vi "Invalid Iteration Error.vi"(7 "error source vi name":string, 8 "error in (no error)":errorcluster, 9 "expected iteration":u64, 10 "actual iteration":u64, 11 "Transfer Group in":refnum<class "Transfer Group.lvclass">) -> (0 "error out":errorcluster, 3 "Transfer Group out":refnum<class "Transfer Group.lvclass">)   [LabVIEW 2017, in "DSF Core.lvlib" / "Transfer Group.lvclass"]
uses:
  Transfer Group.lvclass
  Errors.ctl
  Transfer Group.lvclass/Transfer Group.ctl
  <vilib>/NI/Memory Manager/VIs/New Error Cluster (512B).vi
  <vilib>/NI/Memory Manager/VIs/Write Numeric Scalar to Source (Base10 U64).vi
  Framework/Engine Library Name.vi
  Framework/Framework.lvclass
  <vilib>/NI/Memory Manager/Static Errors.lvlib
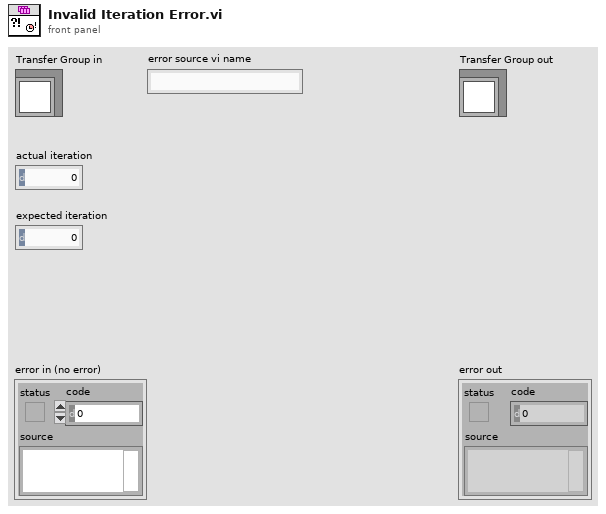
[diagram p1: front panel]
types:
  T1 = typedef "DSF Core.lvlib/Transfer Group.lvclass/Errors.ctl" = enum16{"Return Timeout", "Invalid Iteration"}
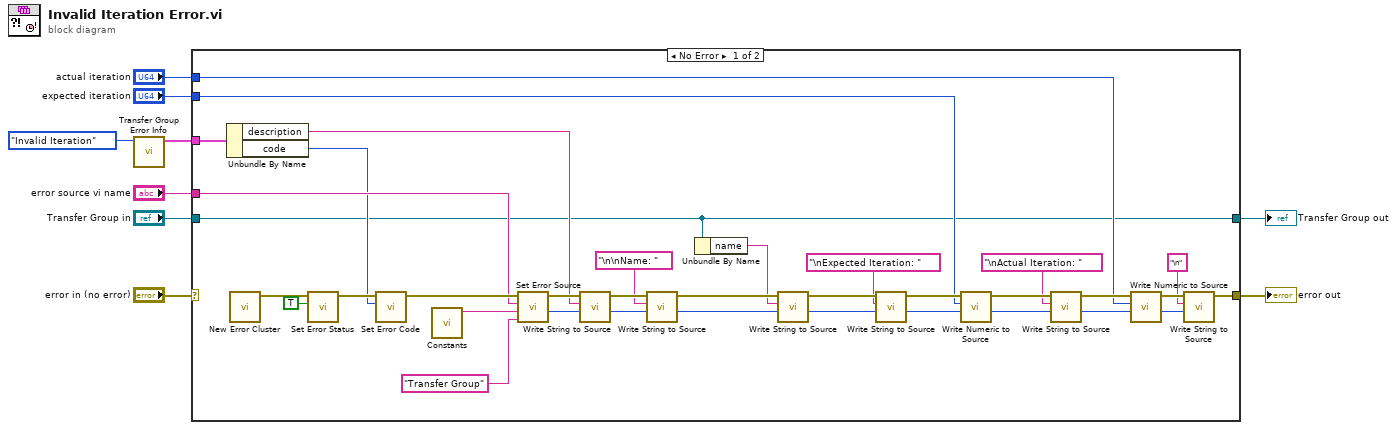
[diagram p0: block diagram]
diagram:
  n1 = call "Transfer Group Error Info.vi"("errors"=Errors."Invalid Iteration") -> ("error info"=w2:cluster{"code":i32, "description":string})  [unwired: 10 in]
  n2 = case shown="No Error" "error in (no error)" {
    selector: "error in (no error)" -> [_ w45]
    tunnel: [w32 w45] -> w8
    tunnel: [w13 w46] -> w7
    tunnel: "Transfer Group in" -> [w13 w46]
    tunnel: "error source vi name" -> [w36 _]
    tunnel: "expected iteration" -> [w21 _]
    tunnel: w2 -> [w28 _]
    tunnel: "actual iteration" -> [w20 _]
    frame No Error {
      n3 = Unbundle By Name(w28) -> ("description"=w22:string, "code"=w27:i32)
      n4 = call-poly <vilib>:"New Error Cluster.vi"() -> ("error out"=w44:errorcluster)  [unwired: 10 in, 1 out]
      n5 = call <vilib>:"Set Error Status.vi"("status (T)"=TRUE, "error in"=w44) -> ("error out"=w43:errorcluster)  [unwired: 9 in]
      n6 = call <vilib>:"Set Error Code.vi"("code"=w27, "error in"=w43) -> ("error out"=w42:errorcluster)  [unwired: 9 in]
      n7 = call-poly "Constants.vi"() -> ("Engine Library Name"=w41:string)  [unwired: 11 in]
      n8 = call <vilib>:"Set Error Source.vi"("class name (\"\")"="Transfer Group" ("Engine Library Name"), "library name (\"\")"=w41, "vi name"=w36, "error in"=w42) -> ("initial offset"=w25:i32, "error out"=w26:errorcluster)  [unwired: 6 in]
      n9 = call <vilib>:"Write String to Source.vi"("offset"=w25, "string"=w22, "error in"=w26) -> ("new offset"=w15:i32, "error out"=w16:errorcluster)  [unwired: 7 in]
      n10 = call <vilib>:"Write String to Source.vi"("offset"=w15, "string"="\n\nName: ", "error in"=w16) -> ("new offset"=w18:i32, "error out"=w19:errorcluster)  [unwired: 7 in]
      n11 = Unbundle By Name(w13) -> ("name"=w17:string)
      n12 = call <vilib>:"Write String to Source.vi"("offset"=w18, "string"=w17, "error in"=w19) -> ("new offset"=w11:i32, "error out"=w12:errorcluster)  [unwired: 7 in]
      n13 = call <vilib>:"Write String to Source.vi"("offset"=w11, "string"="\nExpected Iteration: ", "error in"=w12) -> ("new offset"=w39:i32, "error out"=w40:errorcluster)  [unwired: 7 in]
      n14 = call-poly <vilib>:"Write Numeric to Source.vi"("offset"=w39, "value"=w21, "error in"=w40) -> ("new offset"=w37:i32, "error out"=w38:errorcluster)  [unwired: 7 in]
      n15 = call <vilib>:"Write String to Source.vi"("offset"=w37, "string"="\nActual Iteration: ", "error in"=w38) -> ("new offset"=w34:i32, "error out"=w35:errorcluster)  [unwired: 7 in]
      n16 = call-poly <vilib>:"Write Numeric to Source.vi"("offset"=w34, "value"=w20, "error in"=w35) -> ("new offset"=w31:i32, "error out"=w33:errorcluster)  [unwired: 7 in]
      n17 = call <vilib>:"Write String to Source.vi"("offset"=w31, "string"="\n", "error in"=w33) -> ("error out"=w32:errorcluster)  [unwired: 7 in, 1 out]
    }
    frame Error {
      # "Incoming error. Pass through."
    }
  }
  "error out" <- w8
  "Transfer Group out" <- w7
